vi "GlassSlideLines.vi"() -> ()   [LabVIEW 2017]
uses:
  Shared Components/Gantry Class/Gantry Class.lvclass
  Shared Components/SyringeTool Class/SyringeTool Class.lvclass
  <vilib>/Utility/error.llb/DialogType.ctl
  Shared Components/Config Manager Class/Type Definitions/Camera Enum.ctl
  Shared Components/Vec3d Class/Vec3d Class.lvclass
  Shared Components/Config Manager Class/Type Definitions/Potting Surface Type.ctl
  Shared Components/Gantry Class/Type Definitions/Init_Modes.ctl
  Shared Components/Gantry Class/Type Definitions/Virtual Modes.ctl
  Shared Components/WorkTable Class/WorkTable Class.lvclass
panel:
  out "error out":errorcluster
  out "Image":T1(plugin-control)
  in  "stop":bool
  in  "Config Folder":path=path "C:/Users/Husker/Desktop/gantry/Config"
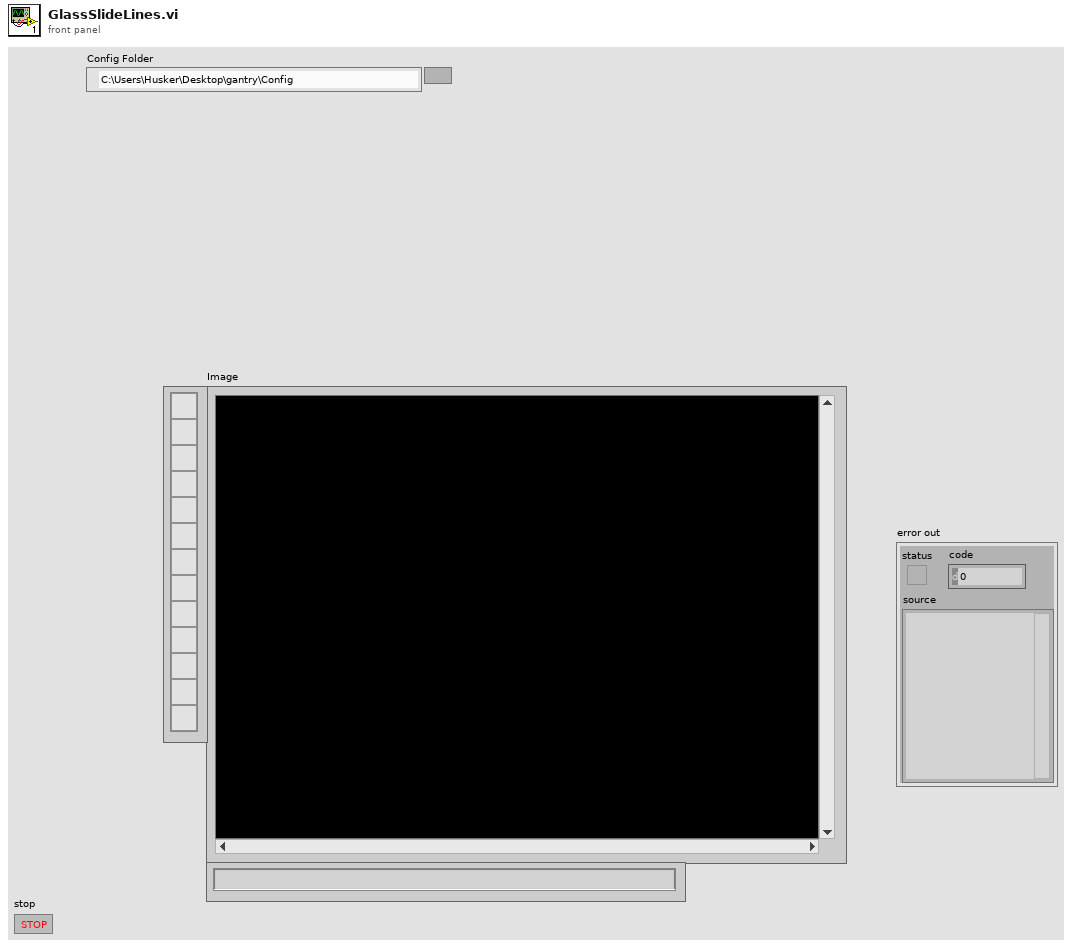
[diagram p1: front panel]
types:
  T1 = typedef "IMAQ Image.ctl" = refnum<image>
  T2 = typedef "Virtual Modes.ctl" = enum16{"Nonvirtual", "Pseudovirtual", "Virtual"}
  T3 = typedef "Init_Modes.ctl" = enum16{"Full", "Robot Only", "Dispenser Only", "Cameras Only", "Robot and Cameras", "Robot and Cameras and Dispenser", "Manifold Only"}
  T4 = typedef "Camera Enum.ctl" = enum16{"GANTRY HEAD", "NEEDLE CALIBRATION X", "NEEDLE CALIBRATION Y", "STAND CAMERA", "SIMRAN WEBCAM"}
  T5 = typedef "DialogType.ctl" = u16
  T6 = typedef "Worktable_Syringe.ctl" = cluster{"Syringe Holder":enum16{"Empty", "Populated", "Calibrated"}, "Mixing Time":timestamp, "Tip Offset":refnum<class "Vec3d Class.lvclass">}
  T7 = typedef "Potting Surface Type.ctl" = enum16{"default", "hdi_edge_pads", "bbm_edge_pads", "address_pads"}
  T8 = typedef "Potting Parameters.ctl" = cluster{"Curing Param A":dbl, "Curing Param B":dbl, "Speed Nominal":dbl, "Time Nominal":dbl, "Turn-on Time":dbl, "Turn-off Time":dbl, "Safe Height Offset":dbl, "Tip Height":dbl, "Width of Line":dbl, "Number of lines":dbl, "Distance between lines":dbl}
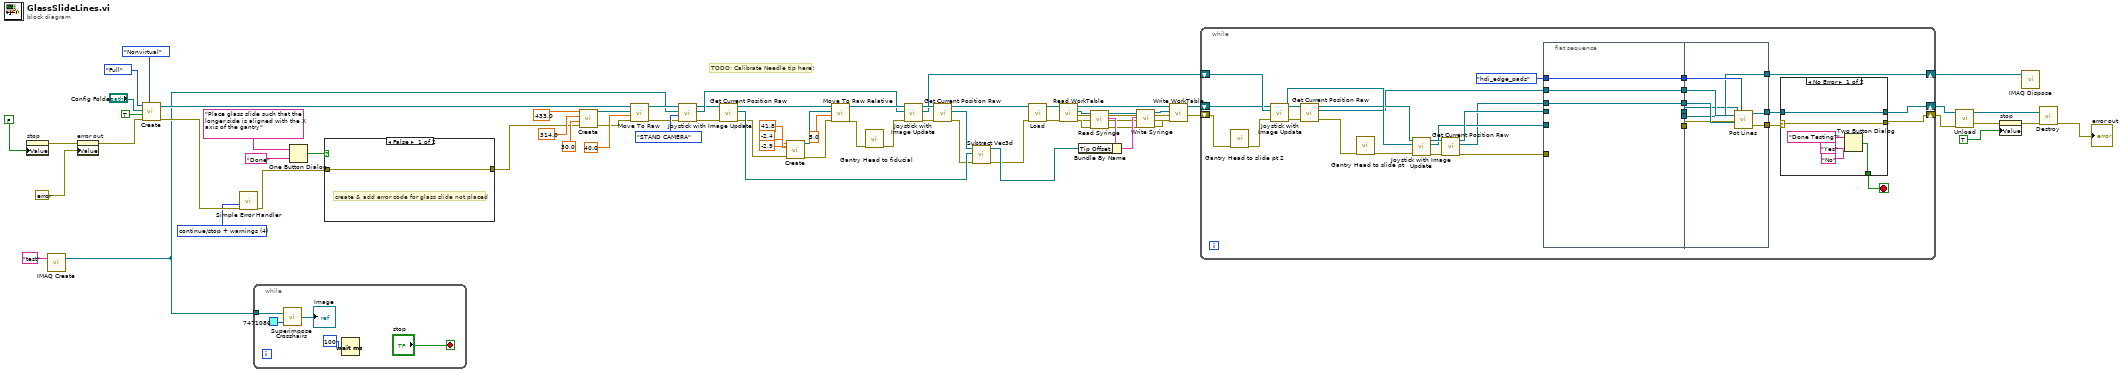
[diagram p0: block diagram]
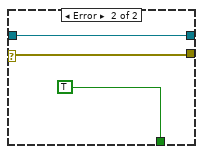
[diagram p2: hidden frame]
diagram:
  w63 = T5 4 items=["no dialog", "OK message", "continue or stop message", "OK message + warnings", "continue/stop + warnings"] ("type of dialog (OK msg:1)")
  # "TODO: Calibrate Needle tip here!"
  n1 = property on="stop" class="Bool (strict)"("Value"=FALSE) -> (error out=w19:errorcluster)  [unwired: 2 in, 1 out]
  n2 = call "IMAQ Create"("Image Name"="test") -> ("New Image"=w32:T1)  [unwired: 4 in, 1 out]
  n3 = property on="error out" class="Clust (strict)"(error in=w19, "Value"=errorcluster {"status"=FALSE, "code"=0, "source"=""} ("error in (no error)")) -> (error out=w16:errorcluster)  [unwired: 1 in, 1 out]
  n4 = call "Create.vi"("Virtual Mode"=Virtual_Modes."Nonvirtual", "error in"=w16, "HOME?"=TRUE, "Config Folder"="Config Folder", "Init Mode"=Init_Modes."Full") -> ("error out"=w65:errorcluster, "Gantry out"=w56:refnum<class "Gantry Class.lvclass">)  [unwired: 5 in]
  n5 = call <vilib>:"Simple Error Handler.vi"("type of dialog (OK msg:1)"=w63, "error in (no error)"=w65) -> ("error out"=w64:errorcluster)  [unwired: 3 in, 4 out]
  n6 = while {
    tunnel: w32 -> [w74]
    stop <- "stop" stop-if-true
    n7 = call "Superimpose Crosshairs.vi"("Grid Line Color"=u32 7471086, "Refnum in"=w74) -> ("Refnum out"=→"Image":T1)
    n8 = Wait (ms)(milliseconds to wait=u32 100) -> ()  [unwired: 1 out]
  }
  n9 = One Button Dialog(message="Place glass slide such that the longer side is aligned with the X axis of the gantry", button name ("OK")="Done" ("F button name (\"Cancel\")")) -> (true=w69:bool)
  n10 = case shown="False" w69 {
    tunnel: w64 -> [w77 w78]
    tunnel: [w77 w78] -> w55
    frame False {
      # "create & add error code for glass slide not placed"
    }
    frame True {
    }
  }
  n11 = call "Create.vi"("error in"=w55, "Z"=30.0, "Y"=314.0, "X"=433.0) -> ("error out"=w60:errorcluster, "Vec3d Class out"=w62:refnum<class "Vec3d Class.lvclass">)  [unwired: 6 in]
  n12 = call-dynamic "Move To Raw.vi"("error in"=w60, "Speed"=40.0, "Destination"=w62, "Gantry in"=w56) -> ("error out"=w34:errorcluster, "Gantry out"=w35:refnum<class "Gantry Class.lvclass">)  [unwired: 6 in]
  n13 = call-dynamic "Joystick with Image Update.vi"("error in (no error)"=w34, "Camera Name"=Camera_Enum."STAND CAMERA", "Image In"=w32, "Gantry Class in"=w35) -> ("error out"=w40:errorcluster, "Image Out"=w43:T1, "Gantry Class out"=w41:refnum<class "Gantry Class.lvclass">)  [unwired: 5 in]
  n14 = call-dynamic "Get Current Position Raw.vi"("error in"=w40, "Gantry in"=w41) -> ("error out"=w37:errorcluster, "Vec3d Class out"=w38:refnum<class "Vec3d Class.lvclass">, "Gantry out"=w39:refnum<class "Gantry Class.lvclass">)  [unwired: 7 in]
  n15 = call "Create.vi"("error in"=w37, "Z"=-2.9, "Y"=-2.4, "X"=41.8) -> ("error out"=w42:errorcluster, "Vec3d Class out"=w47:refnum<class "Vec3d Class.lvclass">)  [unwired: 6 in]
  n16 = call-dynamic "Move To Raw Relative.vi"("error in"=w42, "Speed(mm/s)"=5.0 ("Speed"), "Delta"=w47, "Gantry in"=w39) -> ("error out"=w44:errorcluster, "Gantry out"=w45:refnum<class "Gantry Class.lvclass">)  [unwired: 6 in]
  n17 = call "Gantry Head to fiducial"("error in (no error)"=w44) -> ("error out"=w51:errorcluster)  [unwired: 9 in, 1 out]
  n18 = call-dynamic "Joystick with Image Update.vi"("error in (no error)"=w51, "Image In"=w43, "Gantry Class in"=w45) -> ("error out"=w53:errorcluster, "Image Out"=w1:T1, "Gantry Class out"=w54:refnum<class "Gantry Class.lvclass">)  [unwired: 6 in]
  n19 = call-dynamic "Get Current Position Raw.vi"("error in"=w53, "Gantry in"=w54) -> ("error out"=w30:errorcluster, "Vec3d Class out"=w52:refnum<class "Vec3d Class.lvclass">, "Gantry out"=w2:refnum<class "Gantry Class.lvclass">)  [unwired: 7 in]
  n20 = call "Subtract Vec3d.vi"("error in (no error)"=w30, "Vec3d in 2"=w38, "Vec3d in 1"=w52) -> ("error out"=w3:errorcluster, "Vec3d Class out"=w31:refnum<class "Vec3d Class.lvclass">)  [unwired: 7 in]
  n21 = call "Load.vi"("error in"=w3, "Gantry in"=w2) -> ("error out"=w67:errorcluster, "SyringeTool out"=w68:refnum<class "SyringeTool Class.lvclass">)  [unwired: 8 in]
  n22 = call-dynamic "Read WorkTable.vi"("error in"=w67, "Gantry Class in"=w68) -> ("error out"=w8:errorcluster, "WorkTable Class.lvclass"=w14:refnum<class "WorkTable Class.lvclass">, "Gantry Class out"=w10:refnum<class "SyringeTool Class.lvclass">)  [unwired: 7 in]
  n23 = call "Read Syringe.vi"("error in"=w8, "WorkTable in"=w14) -> ("error out"=w7:errorcluster, "Syringe"=w13:T6, "WorkTable out"=w11:refnum<class "WorkTable Class.lvclass">)  [unwired: 7 in]
  n24 = Bundle By Name(cluster=w13, "Tip Offset"=w31) -> (w12:T6)
  n25 = call-dynamic "Write Syringe.vi"("error in (no error)"=w7, "Syringe"=w12, "WorkTable Class in"=w11) -> ("error out"=w6:errorcluster, "WorkTable Class out"=w9:refnum<class "WorkTable Class.lvclass">)  [unwired: 7 in]
  n26 = call-dynamic "Write WorkTable.vi"("error in (no error)"=w6, "WorkTable Class.lvclass"=w9, "Gantry Class in"=w10) -> ("error out"=w5:errorcluster, "Gantry Class out"=w4:refnum<class "SyringeTool Class.lvclass">)  [unwired: 7 in]
  n27 = while {
    shift-right: [w101] -> w28
    shift-left: w1 -> [w86]
    shift-right: [w96] -> w26
    shift-left: w5 -> [w84]
    shift-right: [w97] -> w27
    shift-left: w4 -> [w85]
    stop <- w107 stop-if-true
    n28 = call "Gantry Head to slide pt 2"("error in (no error)"=w84) -> ("error out"=w88:errorcluster)  [unwired: 9 in, 1 out]
    n29 = call-dynamic "Joystick with Image Update.vi"("error in (no error)"=w88, "Image In"=w86, "Gantry Class in"=w85) -> ("error out"=w87:errorcluster, "Image Out"=w94:T1, "Gantry Class out"=w89:refnum<class "SyringeTool Class.lvclass">)  [unwired: 6 in]
    n30 = call-dynamic "Get Current Position Raw.vi"("error in"=w87, "Gantry in"=w89) -> ("error out"=w95:errorcluster, "Vec3d Class out"=w79:refnum<class "Vec3d Class.lvclass">, "Gantry out"=w93:refnum<class "SyringeTool Class.lvclass">)  [unwired: 7 in]
    n31 = call "Gantry Head to slide pt"("error in (no error)"=w95) -> ("error out"=w91:errorcluster)  [unwired: 9 in, 1 out]
    n32 = call-dynamic "Joystick with Image Update.vi"("error in (no error)"=w91, "Image In"=w94, "Gantry Class in"=w93) -> ("error out"=w90:errorcluster, "Image Out"=w81:T1, "Gantry Class out"=w92:refnum<class "SyringeTool Class.lvclass">)  [unwired: 6 in]
    n33 = call-dynamic "Get Current Position Raw.vi"("error in"=w90, "Gantry in"=w92) -> ("error out"=w82:errorcluster, "Vec3d Class out"=w80:refnum<class "Vec3d Class.lvclass">, "Gantry out"=w83:refnum<class "SyringeTool Class.lvclass">)  [unwired: 7 in]
    n34 = flat-sequence {
      tunnel: w82 -> [_]
      tunnel: Potting_Surface_Type."hdi_edge_pads" ("Potting Surface Type") -> [w112]
      tunnel: w80 -> [w113]
      tunnel: w79 -> [w114]
      tunnel: w83 -> [_]
      tunnel: [w114] -> w106
      tunnel: [w113] -> w105
      tunnel: [w112] -> w104
      tunnel: [w111] -> w103
      tunnel: w81 -> [_]
      tunnel: [w110] -> w102
      tunnel: [w109] -> w100
      tunnel: w106 -> [w123]
      tunnel: w105 -> [w122]
      tunnel: w104 -> [w121]
      tunnel: w103 -> [w120]
      tunnel: [w118] -> w101
      tunnel: w102 -> [w118]
      tunnel: w100 -> [w117]
      tunnel: [w116] -> w99
      tunnel: [w115] -> w98
      frame #0 {
      }
      frame #1 {
        n35 = call-dynamic "Pot Lines.vi"(5:w123, "Potting Surface Type"=w121, "error in"=w120, 9:w122, "SyringeTool in"=w117) -> ("error out"=w115:errorcluster, "SyringeTool out"=w116:refnum<class "SyringeTool Class.lvclass">, "Potting Parameters"=w119:T8)  [unwired: 4 in]
      }
    }
    n36 = case shown="No Error" w98 {
      selector: w98 -> [w125 w132]
      tunnel: [w125 w132] -> w96
      tunnel: [w126 TRUE ("Done Testing?")] -> w107
      tunnel: w99 -> [w124 w130]
      tunnel: [w124 w130] -> w97
      frame No Error {
        n37 = Two Button Dialog(message="Done Testing?", 1:"No" ("F button name (\"Cancel\")"), 2:"Yes" ("T button name (\"OK\")")) -> (T button?=w126:bool)
      }
      frame Error {
      }
    }
  }
  n38 = call "Unload.vi"("error in"=w26, "SyringeTool in"=w27) -> ("error out"=w21:errorcluster, "Gantry out"=w25:refnum<class "Gantry Class.lvclass">)  [unwired: 8 in]
  n39 = property on="stop" class="Bool (strict)"(error in=w21, "Value"=TRUE ("stop")) -> (error out=w20:errorcluster)  [unwired: 1 in, 1 out]
  n40 = call "IMAQ Dispose"("Image"=w28) -> ()  [unwired: 5 in, 1 out]
  n41 = call "Destroy.vi"("error in"=w20, "Gantry Class in"=w25) -> ("error out"=→"error out":errorcluster)  [unwired: 9 in]
